vi "Get Project Item Identation.vi"(9 "Initial Indent":i32, 11 "Item XML String":string) -> (3 "Item Ident":i32)   [LabVIEW 2020, in "LV Project Items Parser.lvlib"]
doc: "Analyzes the item identation level so it can be properly positioned in the Tree Control. The root element should always have an indentation level of 0."
uses:
  LV Project Items Parser.lvlib
  <vilib>/regexp/Match Regular Expression.xnode
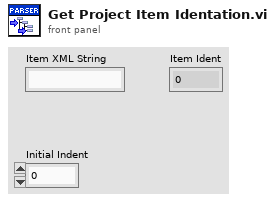
[diagram p1: front panel]
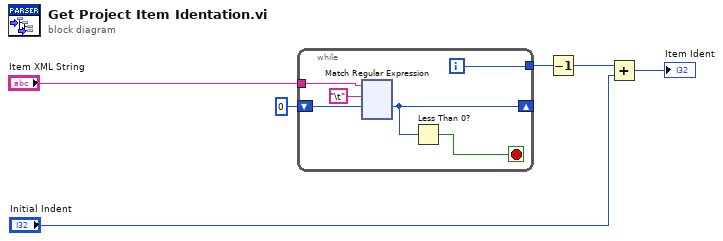
[diagram p0: block diagram]
diagram:
  n1 = while {
    tunnel: [w8] -> w3
    shift-right: [w10] -> _
    shift-left: 0 -> [w9]
    tunnel: "Item XML String" -> [w7]
    i -> [w8]
    stop <- w12 stop-if-true
    n2 = xnode "Match Regular Expression"("input string"=w7, "regular expression"="\t", "offset (0)"=w9) -> ("offset past match"=w10:i32)  [unwired: 3 in, 4 out]
    n3 = Less Than 0?(x=w10) -> (x < 0?=w12:bool)
  }
  n4 = Decrement(x=w3) -> (x-1=w6:i32)
  n5 = Add(x=w6, y="Initial Indent") -> (x+y=→"Item Ident":i32)
